vi "Read Calibration Routine.vi"(8 "error in":errorcluster, 11 "Calibration Actor in":refnum<class "Calibration Actor.lvclass">) -> (0 "error out":errorcluster, 1 "Vals":string[](array[string]), 2 "tags":string[](array[string]), 3 "Calibration Actor out":refnum<class "Calibration Actor.lvclass">)   [LabVIEW 2014, in "Calibration.lvlib" / "Calibration Actor.lvclass"]
doc: "Parse the calibration file that is loaded and load the steps as necessary."
uses:
  Calibration Actor.lvclass
  reusable/Sequence/SEQ/SEQ.lvclass
  Common/Set cycle state/Set cycle state STEP.lvclass
  <vilib>/ActorFramework/Actor/Actor.lvclass/Actor.ctl
  Calibration Actor.lvclass/Calibration Actor.ctl
  reusable/Sequence/STEPS/STEP.lvclass/STEP.ctl
  Common/Wait/Wait STEP.lvclass
  Common/O2 Valve/O2 Valve STEP.lvclass
  reusable/Sequence/STEPS/STEP.lvclass
  Common/O2 Flow Rate/O2 Flow Rate STEP.lvclass
  Common/Speaker/Speaker STEP.lvclass
  Common/Filter/Filter Step/Filter STEP.lvclass
  Common/O3 Level/O3 Level STEP.lvclass
  Common/O3 Generator Power/O3 Generator Power STEP.lvclass
  <vilib>/regexp/Match Regular Expression.xnode
  <vilib>/ActorFramework/Actor/Actor.lvclass
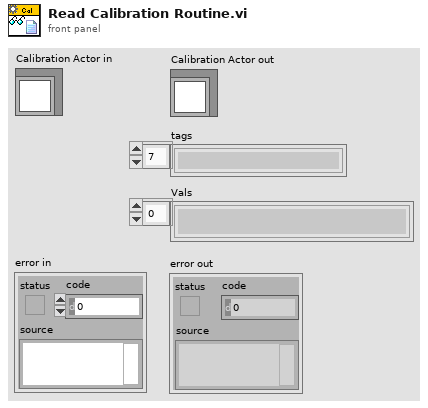
[diagram p1: front panel]
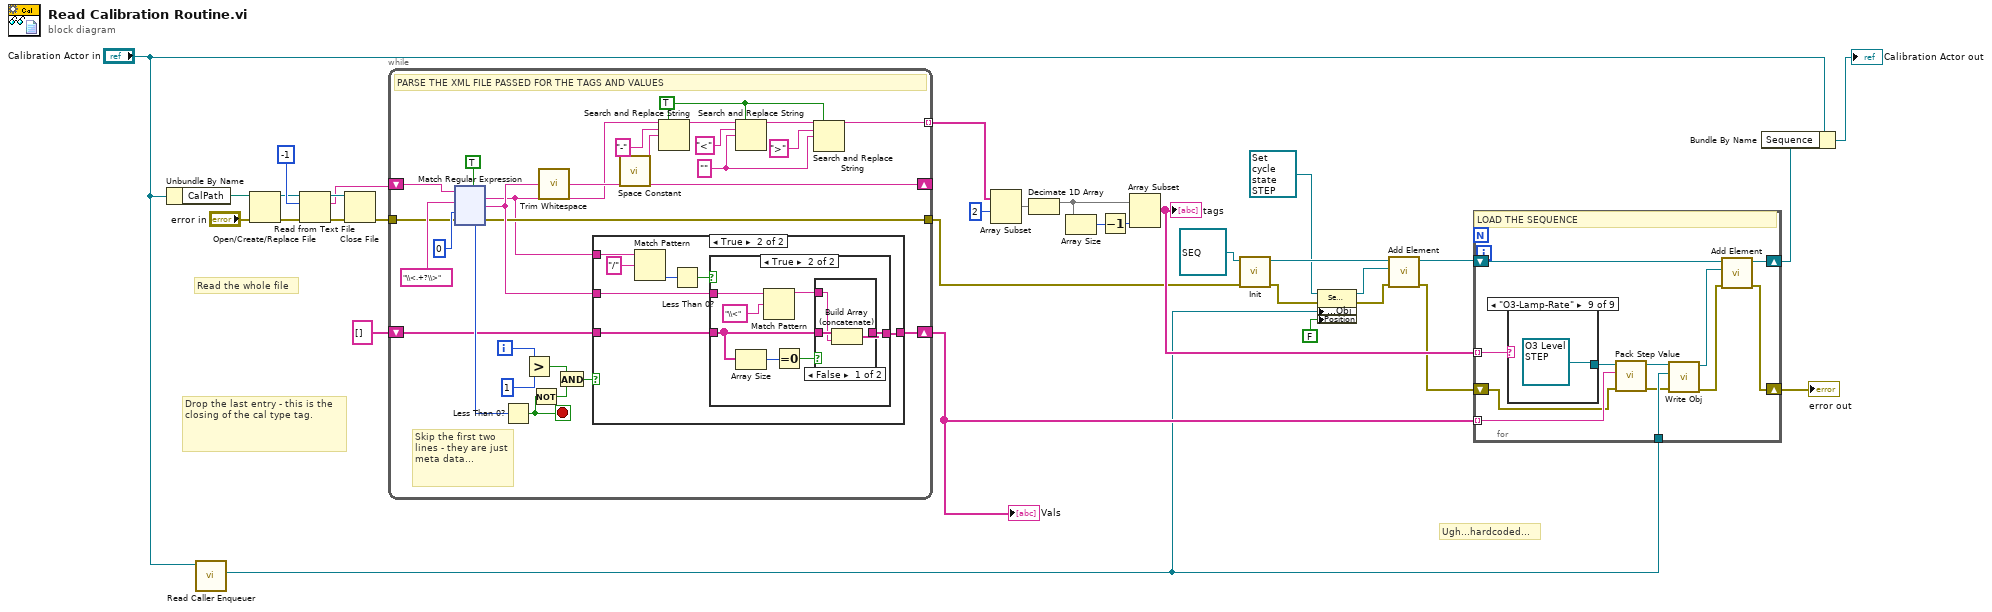
[diagram p0: block diagram]
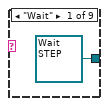
[diagram p2: hidden frame]
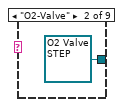
[diagram p3: hidden frame]
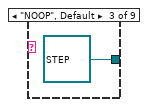
[diagram p4: hidden frame]
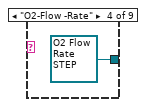
[diagram p5: hidden frame]
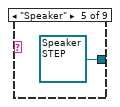
[diagram p6: hidden frame]
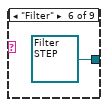
[diagram p7: hidden frame]
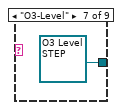
[diagram p8: hidden frame]
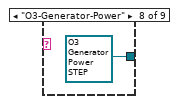
[diagram p9: hidden frame]
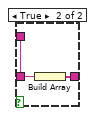
[diagram p12: hidden frame]
diagram:
  # "Ugh...hardcoded..."
  # "Read the whole file"
  # "Drop the last entry - this is the closing of the cal type tag."
  n1 = Unbundle By Name("Calibration Actor in") -> ("CalPath"=w1:path)
  n2 = call <vilib>:"Read Caller Enqueuer.vi"("Actor"="Calibration Actor in") -> ("Caller Enqueuer"=w7:refnum<class "Message Enqueuer.lvclass">)  [unwired: 10 in]
  n3 = Open/Create/Replace File(file path (use dialog)=w1, error in="error in") -> (refnum out=w31:refnum<file>, error out=w30:errorcluster)  [unwired: 4 in, 1 out]
  n4 = Read from Text File(file (use dialog)=w31, count=-1, error in=w30) -> (refnum out=w29:refnum<file>, text=w28:string, error out=w21:errorcluster)  [unwired: 1 in, 1 out]
  n5 = Close File(refnum=w29, error in=w21) -> (error out=w20:errorcluster)  [unwired: 1 out]
  n6 = while {
    shift-right: [w59] -> _
    shift-left: w28 -> [w58]
    shift-right: [w48] -> w12
    shift-left: string[] [] -> [w49]
    tunnel: w20 -> [w45]
    tunnel: [w44] -> w5
    tunnel: [w37] -> w19 mode=indexing
    i -> [w53]
    stop <- w46 stop-if-true
    w34 = "" ("replace string (\"\")")
    w36 = TRUE ("ignore case? (F)")
    # "Skip the first two lines - they are just meta data..."
    # "PARSE THE XML FILE PASSED FOR THE TAGS AND VALUES"
    n7 = xnode "Match Regular Expression"("input string"=w58, "regular expression"="\\<.+?\\>", "offset (0)"=0, "error in"=w45, "multiline? (F)"=TRUE) -> ("whole match"=w41:string, "after match"=w55:string, "offset past match"=w56:i32, "error out"=w44:errorcluster)  [unwired: 1 in, 1 out]
    n8 = Less Than 0?(x=w56) -> (x < 0?=w46:bool)
    n9 = Greater?(x=w53, y=1) -> (0:w51:bool)
    n10 = Not(x=w46) -> (.not. x?=w47:bool)
    n11 = call <vilib>:"Trim Whitespace.vi"("string"=w55) -> ("trimmed string"=w59:string)  [unwired: 1 in]
    n12 = And(x=w51, y=w47) -> (x .and. y?=w50:bool)
    n13 = case shown="True" w50 {
      tunnel: w41 -> [_ w68]
      tunnel: w55 -> [_ w64]
      tunnel: w49 -> [w61 w63]
      tunnel: [w61 w62] -> w48
      frame False {
      }
      frame True {
        n14 = Match Pattern(string=w68, regular expression="/") -> (offset past match=w66:i32)  [unwired: 1 in, 3 out]
        n15 = Less Than 0?(x=w66) -> (x < 0?=w65:bool)
        n16 = case shown="True" w65 {
          tunnel: w64 -> [_ w76]
          tunnel: w63 -> [w69 w71]
          tunnel: [w69 w72] -> w62
          frame False {
          }
          frame True {
            n17 = Array Size(array=w71) -> (size(s)=w73:i32)
            n18 = Match Pattern(string=w76, regular expression="\\<") -> (before substring=w70:string)  [unwired: 1 in, 3 out]
            n19 = Equal To 0?(x=w73) -> (x = 0?=w74:bool)
            n20 = case shown="False" w74 {
              tunnel: w70 -> [w77 w81]
              tunnel: [w78 w80] -> w72
              tunnel: w71 -> [w79 _]
              frame False {
                n21 = Build Array (concatenate)(w79, w77) -> (w78:string[])
              }
              frame True {
                n22 = Build Array(w81) -> (w80:string[])
              }
            }
          }
        }
      }
    }
    n23 = call <vilib>:"Space Constant.vi"() -> ("String"=w42:string)
    n24 = Search and Replace String(replace all?=w36, input string=w41, search string="-", replace string=w42) -> (result string=w40:string)  [unwired: 4 in, 3 out]
    n25 = Search and Replace String(replace all?=w36, input string=w40, search string="<", replace string=w34) -> (result string=w38:string)  [unwired: 4 in, 3 out]
    n26 = Search and Replace String(replace all?=w36, input string=w38, search string=">", replace string=w34) -> (result string=w37:string)  [unwired: 4 in, 3 out]
  }
  "Vals" <- w12
  n27 = Array Subset(array=w19, index=2) -> (w25:string[])  [unwired: 1 in]
  n28 = Decimate 1D Array(w25) -> (w24:string[])  [unwired: 1 out]
  n29 = Array Size(array=w24) -> (size(s)=w23:i32)
  n30 = Decrement(x=w23) -> (x-1=w22:i32)
  n31 = Array Subset(array=w24, length=w22) -> (w18:string[])  [unwired: 1 in]
  "tags" <- w18
  n32 = call-dynamic "Init.vi"("error in"=w5, "SEQ in"=refnum<class "SEQ.lvclass"> refnum ("Sequence Composition:SEQ")) -> ("error out"=w4:errorcluster, "SEQ out"=w11:refnum<class "SEQ.lvclass">)  [unwired: 8 in]
  n33 = property class="Set cycle state STEP.lvclass"(reference=refnum<class "Set cycle state STEP.lvclass"> refnum ("Set cycle state STEP.lvclass"), error in=w4, "Accessors:Obj"=w7, "Position"=FALSE) -> (reference out=w6:refnum<class "Set cycle state STEP.lvclass">, error out=w3:errorcluster)
  n34 = call "Add Element.vi"("error in"=w3, "STEP"=w6, "SEQ in"=w11) -> ("error out"=w2:errorcluster, "SEQ out"=w10:refnum<class "SEQ.lvclass">)  [unwired: 7 in]
  n35 = for {
    tunnel: w18 -> [w207] mode=indexing
    tunnel: w12 -> [w205] mode=indexing
    tunnel: w7 -> [w204]
    shift-right: [w196] -> w13
    shift-left: w2 -> [w201]
    shift-right: [w198] -> w14
    shift-left: w10 -> [w199]
    # "LOAD THE SEQUENCE"
    n36 = case shown="\"O3-Lamp-Rate\"" w207 {
      tunnel: [refnum<class "Wait STEP.lvclass"> refnum ("Wait") refnum<class "O2 Valve STEP.lvclass"> refnum ("O2 Valve") refnum<class "STEP.lvclass"> refnum ("Sequence Composition:STEP.lvclass") refnum<class "O2 Flow Rate STEP.lvclass"> refnum ("O2 Flow Rate") refnum<class "Speaker STEP.lvclass"> refnum ("Speaker") refnum<class "Filter STEP.lvclass"> refnum ("Filter") refnum<class "O3 Level STEP.lvclass"> refnum ("O3 Level") refnum<class "O3 Generator Power STEP.lvclass"> refnum ("O3 Generator Power") refnum<class "O3 Level STEP.lvclass"> refnum ("O3 Level")] -> w206
      frame "Wait" {
      }
      frame "O2-Valve" {
      }
      frame "NOOP", Default {
      }
      frame "O2-Flow -Rate" {
      }
      frame "Speaker" {
      }
      frame "Filter" {
      }
      frame "O3-Level" {
      }
      frame "O3-Generator-Power" {
      }
      frame "O3-Lamp-Rate" {
      }
    }
    n37 = call-dynamic "Pack Step Value.vi"("error in (no error)"=w201, "Value"=w205, "STEP in"=w206) -> ("error out"=w202:errorcluster, "STEP out"=w203:refnum<class "STEP.lvclass">)  [unwired: 7 in]
    n38 = call "Write Obj.vi"("error in (no error)"=w202, "Obj"=w204, "STEP in"=w203) -> ("error out"=w197:errorcluster, "STEP out"=w200:refnum<class "STEP.lvclass">)  [unwired: 7 in]
    n39 = call "Add Element.vi"("error in"=w197, "STEP"=w200, "SEQ in"=w199) -> ("error out"=w196:errorcluster, "SEQ out"=w198:refnum<class "SEQ.lvclass">)  [unwired: 7 in]
  }
  "error out" <- w13
  n40 = Bundle By Name(cluster="Calibration Actor in", "Sequence"=w14) -> (→"Calibration Actor out":refnum<class "Calibration Actor.lvclass">)
